vi "Add Monitoring Channels.vi"(8 "error in (no error)":errorcluster, 10 "Framework Configuration":refnum<class "Framework Configuration.lvclass">, 11 "Item Ref in":T1 format="%.0x") -> (0 "error out":errorcluster, 3 "Item Ref out":T1 format="%.0x")   [LabVIEW 2024, in "DSF System Explorer.lvlib"]
uses:
  DSF System Explorer.lvlib
  <vilib>/NI VeriStand/Custom Device API/Custom Device Channel.ctl
  <vilib>/NI VeriStand/Custom Device API/Custom Device Channel Type.ctl
  Includes/DSF Core.lvlibp/Classes/Configuration/Core/Framework/Framework Configuration.lvclass
  <vilib>/NI VeriStand/Custom Device API/Custom Device API.lvlib
  Shared/DSF Shared.lvlib
  <vilib>/NI VeriStand/Custom Device API/Custom Device Item Ref.ctl
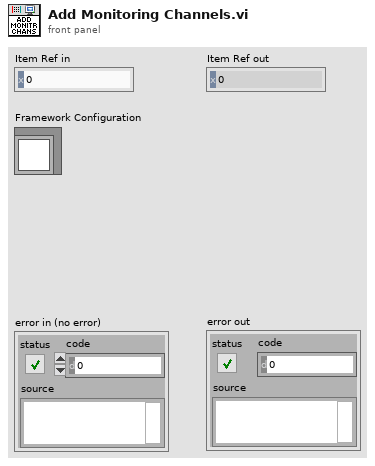
[diagram p1: front panel]
types:
  T1 = typedef "Custom Device API.lvlib/Custom Device Item Ref.ctl" = u64
  T2 = typedef "Custom Device API.lvlib/Custom Device Channel.ctl" = cluster{"Type":T3, "Units":string, "Default Value":dbl, "Faultable":bool, "Scalable":bool}
  T3 = typedef "Custom Device API.lvlib/Custom Device Channel Type.ctl" = enum16{"Input", "Output"}
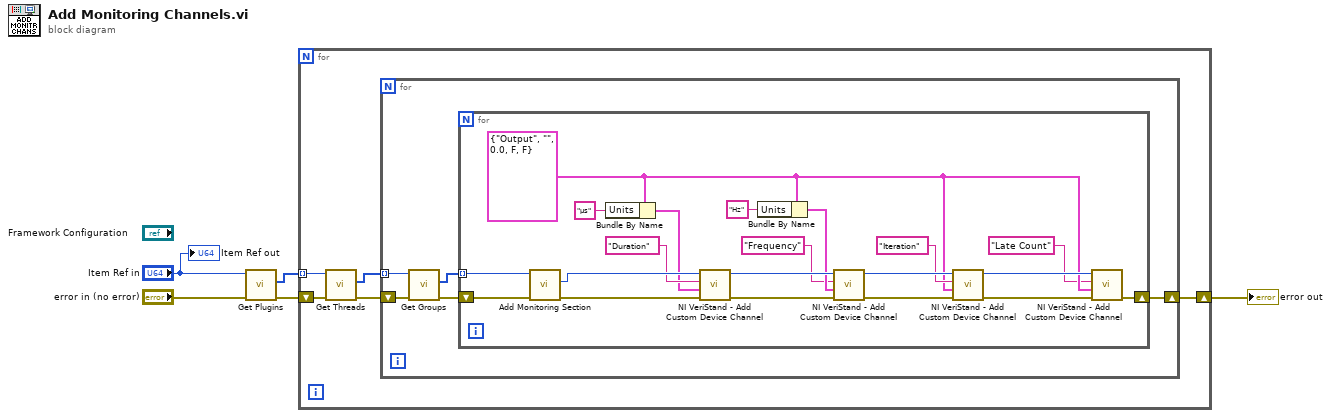
[diagram p0: block diagram]
diagram:
  n1 = call "Get Plugins.vi"("error in (no error)"="error in (no error)", "Item Ref in"="Item Ref in") -> ("error out"=w3:errorcluster, "Plugin refs"=w1:T1[])  [unwired: 7 in, 1 out]
  n2 = for {
    tunnel: w1 -> [w8] mode=indexing
    shift-right: [w10] -> w4
    shift-left: w3 -> [w9]
    n3 = call "Get Threads.vi"("error in (no error)"=w9, "Item Ref in"=w8) -> ("error out"=w7:errorcluster, "Plugin refs"=w6:T1[])  [unwired: 7 in, 1 out]
    n4 = for {
      tunnel: w6 -> [w13] mode=indexing
      shift-right: [w15] -> w10
      shift-left: w7 -> [w14]
      n5 = call "Get Groups.vi"("error in (no error)"=w14, "Plugin Ref in"=w13) -> ("error out"=w12:errorcluster, "Group refs"=w11:T1[])  [unwired: 7 in, 1 out]
      n6 = for {
        tunnel: w11 -> [w20] mode=indexing
        shift-right: [w33] -> w15
        shift-left: w12 -> [w21]
        w23 = T2 {"Type"=enum."Output", "Units"="", "Default Value"=0.0, "Faultable"=FALSE, "Scalable"=FALSE} ("Channel")
        n7 = call "Add Monitoring Section.vi"("error in (no error)"=w21, "Item Ref in"=w20) -> ("error out"=w19:errorcluster, "Performance Section Ptr"=w18:T1)  [unwired: 7 in, 1 out]
        n8 = Bundle By Name(cluster=w23, "Units"="µs" ("Section Name")) -> (w16:T2)
        n9 = call <vilib>:"NI VeriStand - Add Custom Device Channel.vi"("error in (no error)"=w19, "Channel"=w16, "Channel Name"="Duration" ("Section Name"), "Parent Ref in"=w18) -> ("error out"=w32:errorcluster, "Parent Ref out"=w31:T1)  [unwired: 4 in, 2 out]
        n10 = Bundle By Name(cluster=w23, "Units"="Hz") -> (w26:T2)
        n11 = call <vilib>:"NI VeriStand - Add Custom Device Channel.vi"("error in (no error)"=w32, "Channel"=w26, "Channel Name"="Frequency" ("Section Name"), "Parent Ref in"=w31) -> ("error out"=w30:errorcluster, "Parent Ref out"=w29:T1)  [unwired: 4 in, 2 out]
        n12 = call <vilib>:"NI VeriStand - Add Custom Device Channel.vi"("error in (no error)"=w30, "Channel"=w23, "Channel Name"="Iteration" ("Section Name"), "Parent Ref in"=w29) -> ("error out"=w28:errorcluster, "Parent Ref out"=w27:T1)  [unwired: 4 in, 2 out]
        n13 = call <vilib>:"NI VeriStand - Add Custom Device Channel.vi"("error in (no error)"=w28, "Channel"=w23, "Channel Name"="Late Count" ("Section Name"), "Parent Ref in"=w27) -> ("error out"=w33:errorcluster)  [unwired: 4 in, 3 out]
      }
    }
  }
  "error out" <- w4
  "Item Ref out" <- "Item Ref in"
